vi "CSM - State Dashboard - DebugTool.vi"() -> ()   [LabVIEW 2017]
doc: "Real-time status dashboard for the entire CSM program module."
uses:
  user.lib/_NEVSTOP/Communicable State Machine(CSM)/_Support/Typedef/_CSM_GlobalLog_MSG.ctl
  user.lib/_NEVSTOP/Communicable State Machine(CSM)/_Support/Typedef/_CSM_Response Source Message.ctl
  user.lib/_NEVSTOP/Communicable State Machine(CSM)/_Support/Typedef/_CSM_GlobalLog_MSG_TYPE.ctl
  c0297aac-4a47-44f3-ae53-0a8cf90c2ba3.vi
  62af1497-def4-443f-94d3-5d00758f2f69.vi
  <vilib>/Utility/config.llb/Close Config Data.vi
  <vilib>/Utility/config.llb/Write Key.vi
  <vilib>/Utility/config.llb/Write Key (Double).vi
  <vilib>/Utility/config.llb/Write Key (I32).vi
  <vilib>/Utility/config.llb/Write Key (String).vi
  user.lib/_NEVSTOP/Communicable State Machine(CSM)/_csmHelper/lvcsmFile/Path to lvcsm String.vi
  <vilib>/Utility/config.llb/Remove Key.vi
  <vilib>/Utility/config.llb/Get Key Names.vi
  <vilib>/Utility/Data Type/Get Type Information.vi
  <vilib>/Utility/Data Type/Get Array Information.vi
  <vilib>/Utility/config.llb/Write Key (Boolean).vi
  <vilib>/Utility/config.llb/Open Config Data.vi
  user.lib/_NEVSTOP/Communicable State Machine(CSM)/_csmHelper/lvcsmFile/lvcsm File Path.vi
  user.lib/_NEVSTOP/Communicable State Machine(CSM)/_csmHelper/lvcsmFile/_Array of VData to VCluster.vi
  <vilib>/Utility/config.llb/Read Key.vi
  <vilib>/Utility/config.llb/Read Key (Double).vi
  <vilib>/Utility/config.llb/Read Key (I32).vi
  user.lib/_NEVSTOP/Communicable State Machine(CSM)/_csmHelper/lvcsmFile/lvcsm String to Path.vi
  <vilib>/Utility/config.llb/Read Key (String).vi
  <vilib>/Utility/config.llb/Read Key (Boolean).vi
  user.lib/_NEVSTOP/Communicable State Machine(CSM)/_Polymophic/Add State(s) to Queue By BOOL(Element).vi
  user.lib/_NEVSTOP/Communicable State Machine(CSM)/_tool/_ui/csm-ui-support.lvlib
  user.lib/_NEVSTOP/Communicable State Machine(CSM)/Communicable State Machine.lvlib
panel:
  in  "ColNum:":i16=4 min=2 max=10 step=1
  in  "RowNum:":i16=2 min=2 max=10 step=1
  in  "Clear CSM":bool
  out "Dashboard":T1(array[cluster])
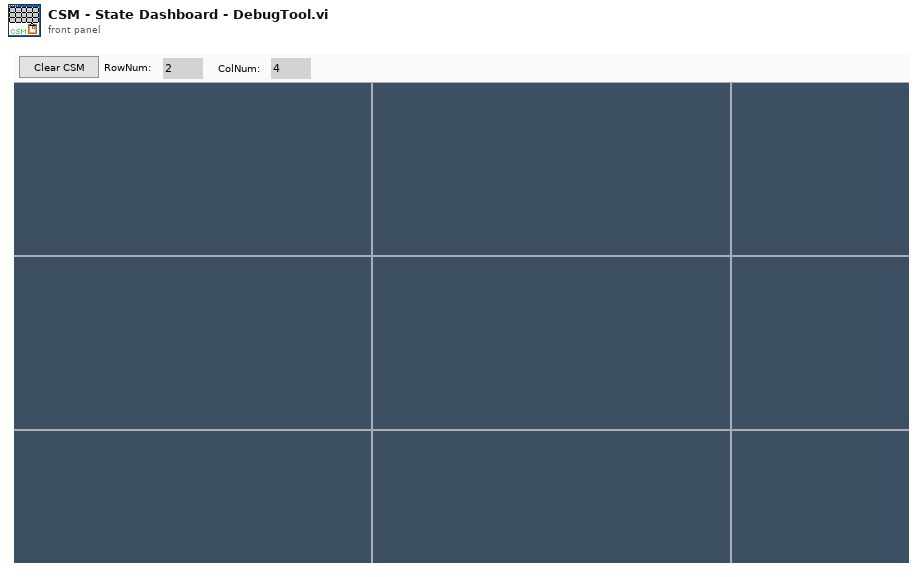
[diagram p1: front panel]
types:
  T1 = cluster{"Label":string, "Value":string, "String":string}[][]
  T2 = enum32{"Invalid", "Standard", "Closed", "Hidden", "Minimized", "Maximized"}
  T3 = enum32{"invalid app kind", "Development System", "Run Time System", "Student Edition", "Embedded LabVIEW", "Evaluation", "Custom"}
  T4 = typedef "Communicable State Machine.lvlib/_CSM_GlobalLog_MSG.ctl" = cluster{"Name (\"\" to Use UUID)":string, "Current State":string, "Arguments":string, "Source Message":T5, "Source Module":string, "Complete(T)/Start(F)":bool, "LogType":T6, "Time Stamp":timestamp}
  T5 = typedef "Communicable State Machine.lvlib/_CSM_Response Source Message.ctl" = cluster{"‘State":string, "’Arguments":string, "’Error":errorcluster}
  T6 = typedef "Communicable State Machine.lvlib/_CSM_GlobalLog_MSG_TYPE.ctl" = enum16{"User Log", "State Change", "Status", "Interrupt", "Register", "Unregister", "Error Log", "Module Created", "Module Destroyed"}
  T7 = cluster{"Label":string, "Value":string, "String":string}
  T8 = cluster{"Core":cluster{"Current VI Reference":refnum<vi>, "Close Panel on Exit?":bool}, "Global-DataTable":string[][], "Configuration":cluster{"NumRows":i16, "NumCols":i16}, "Global Log Event":refnum<user-event>, "Log":T4}
  T9 = cluster{"Current VI Reference":refnum<vi>, "Close Panel on Exit?":bool}
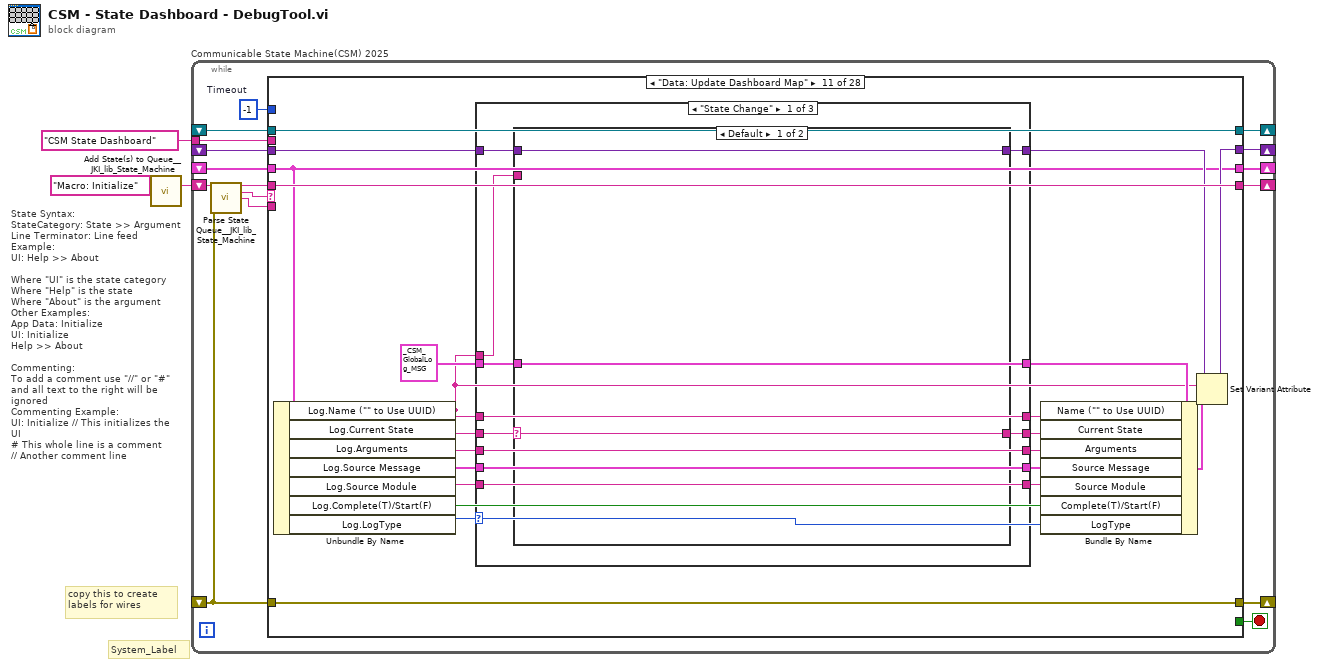
[diagram p0: block diagram]
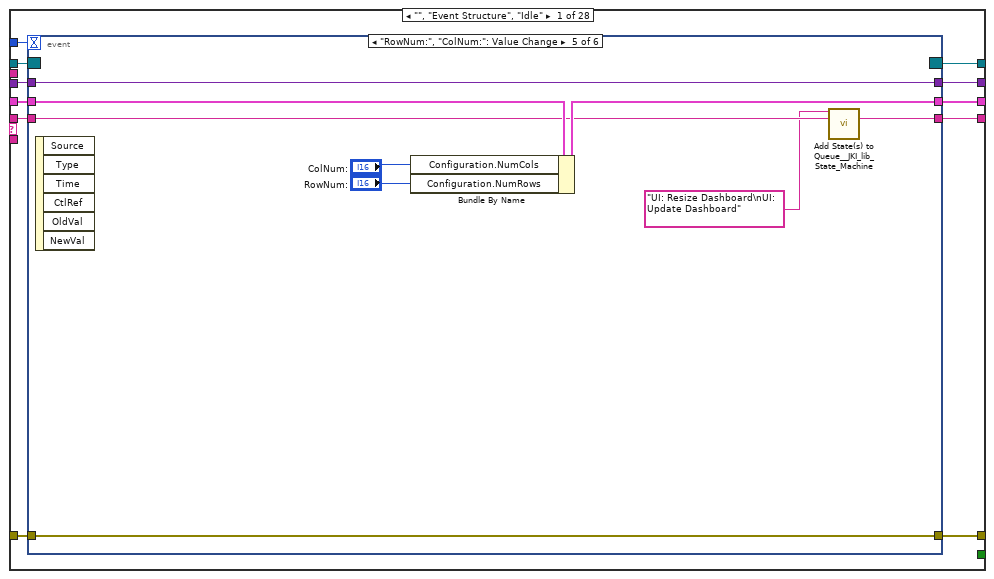
[diagram p2: hidden frame]
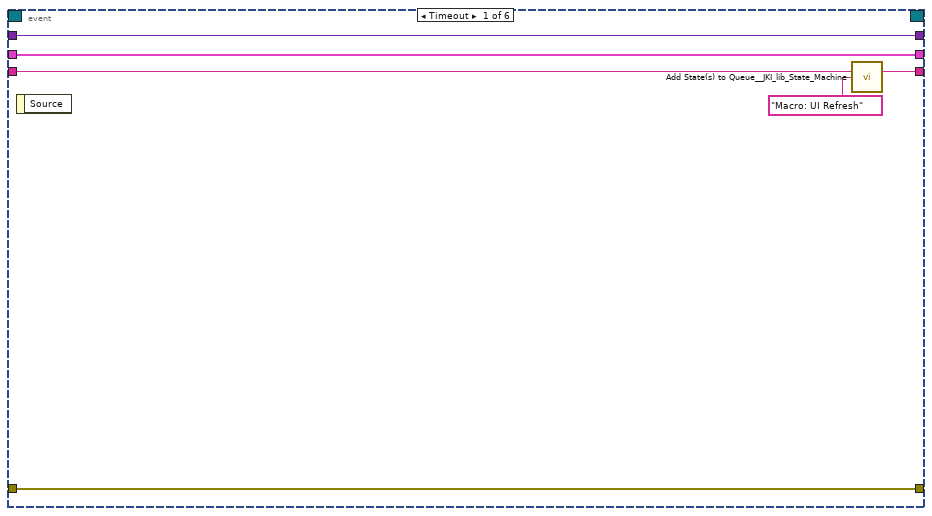
[diagram p3: hidden frame]
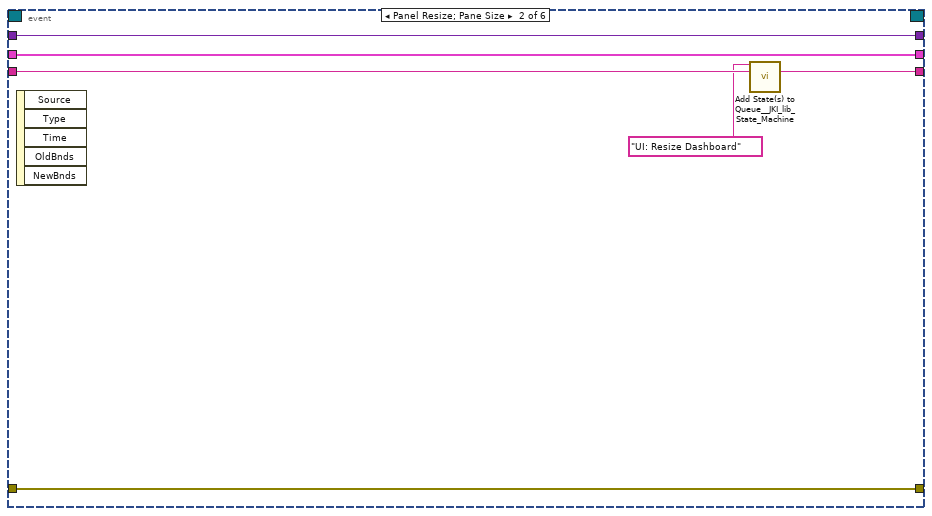
[diagram p4: hidden frame]
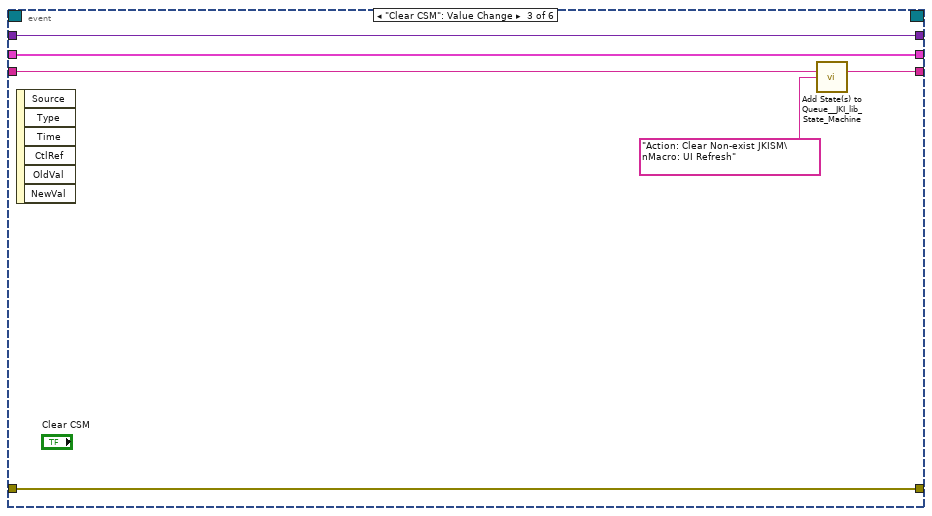
[diagram p5: hidden frame]
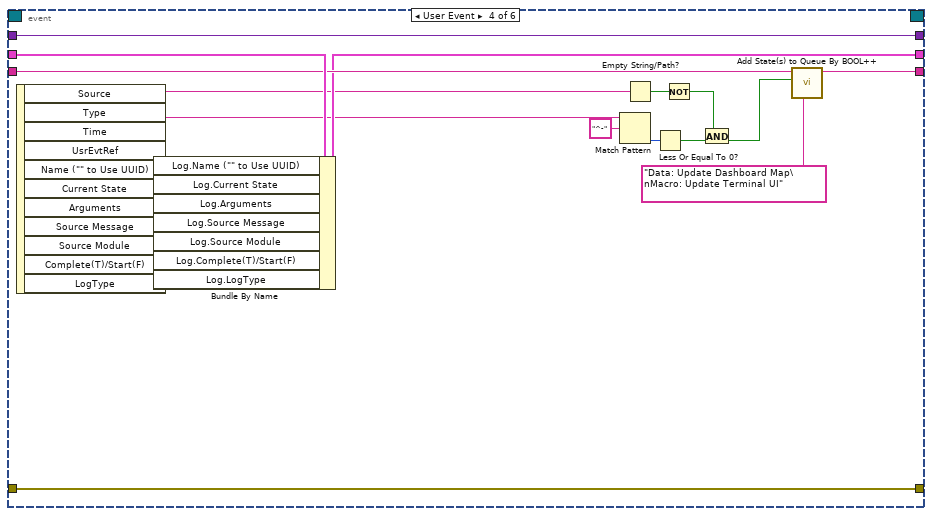
[diagram p6: hidden frame]
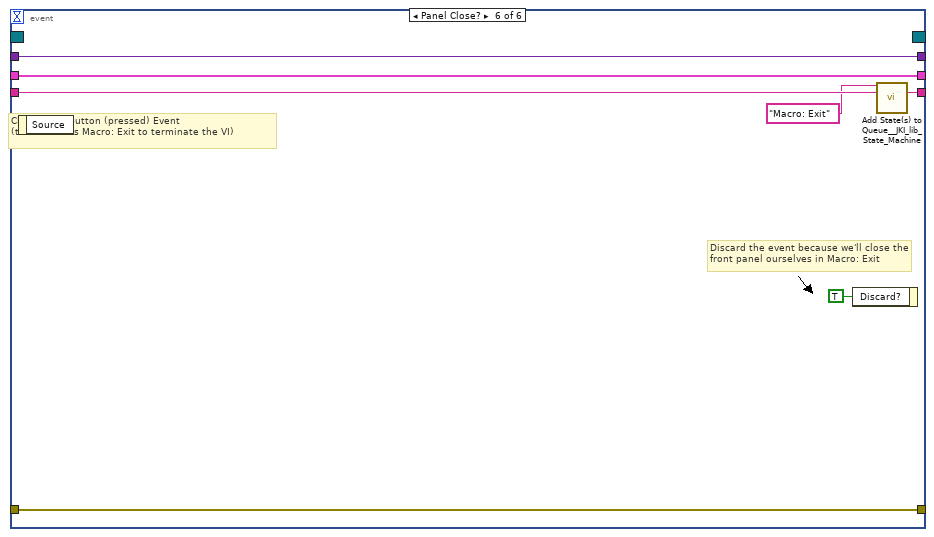
[diagram p7: hidden frame]
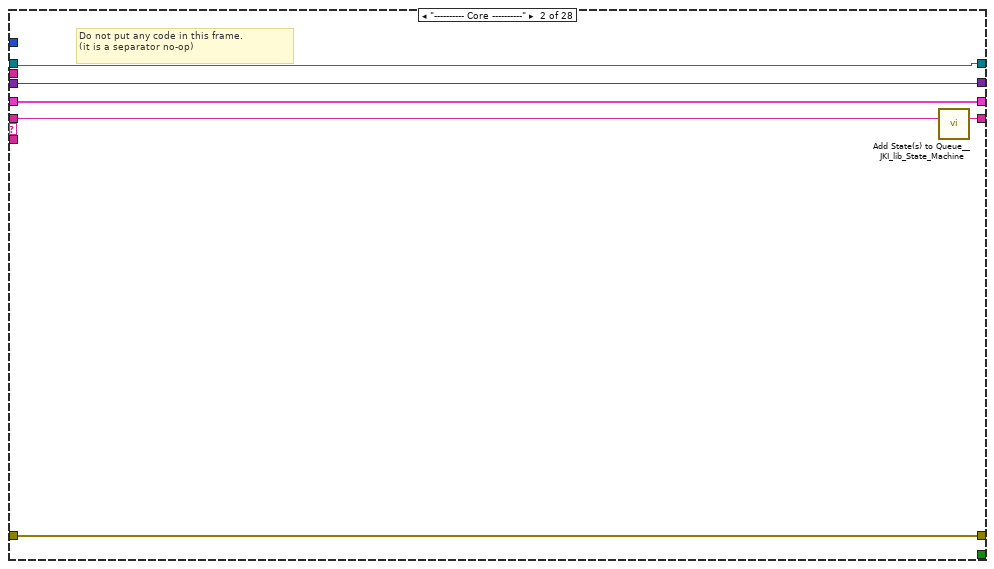
[diagram p8: hidden frame]
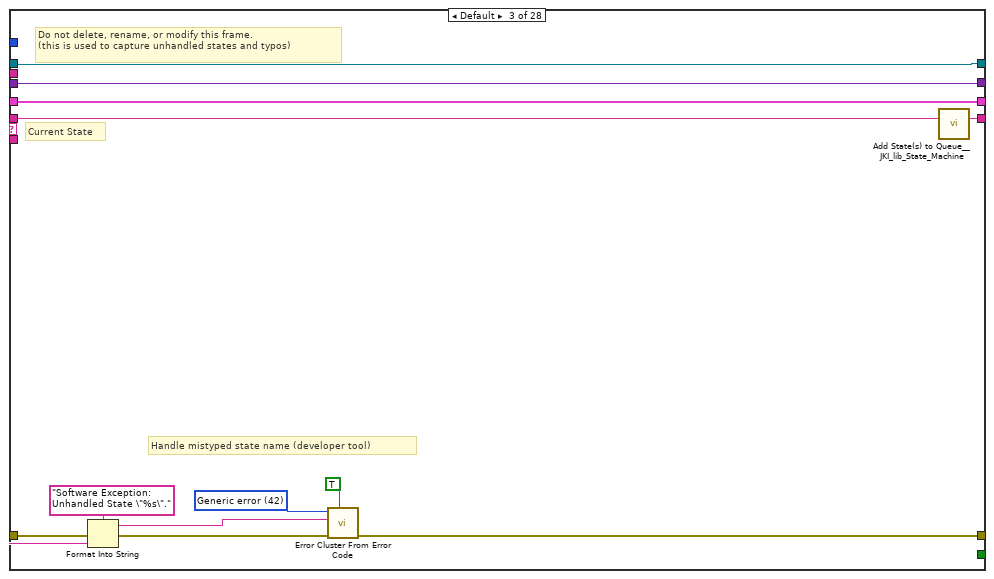
[diagram p9: hidden frame]
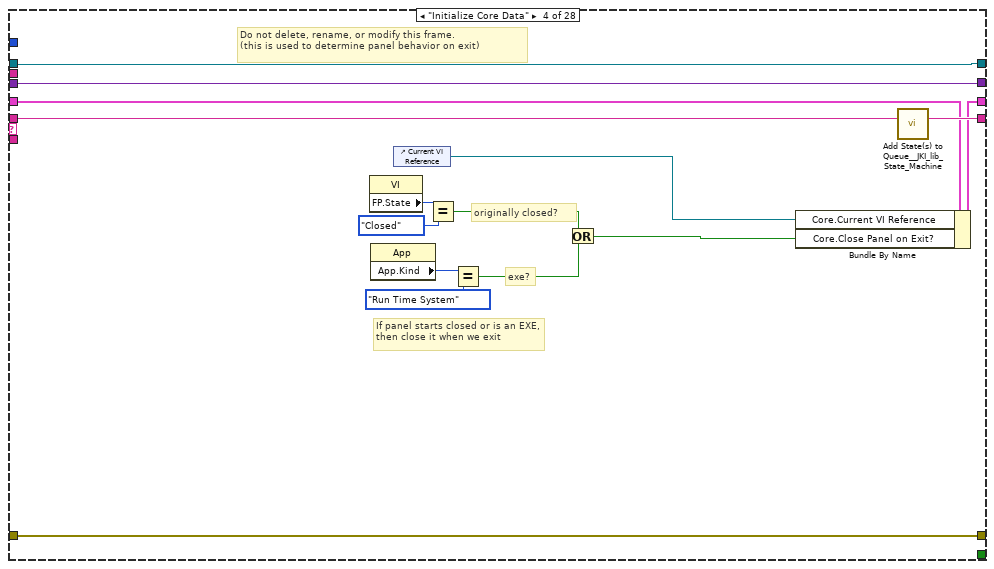
[diagram p10: hidden frame]
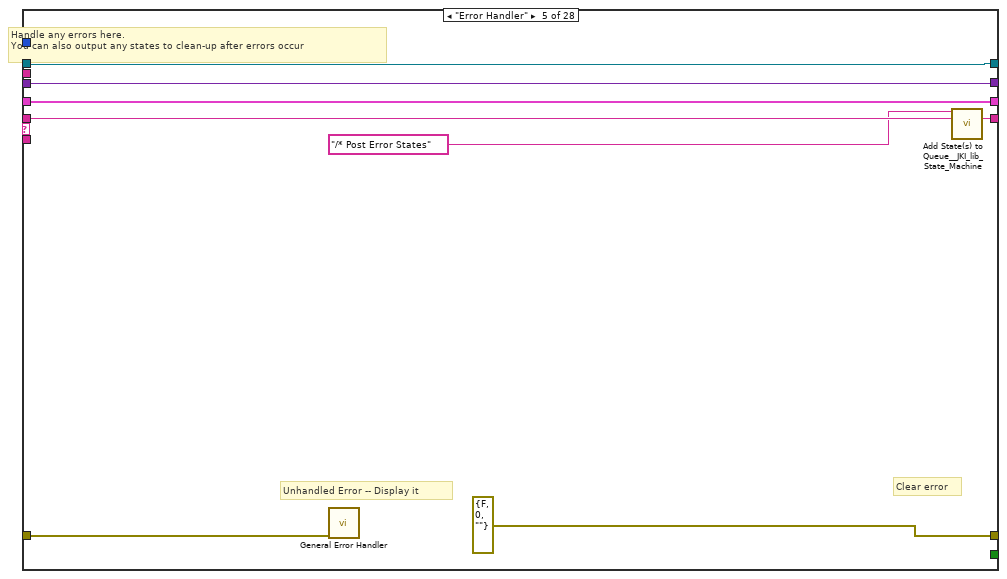
[diagram p11: hidden frame]
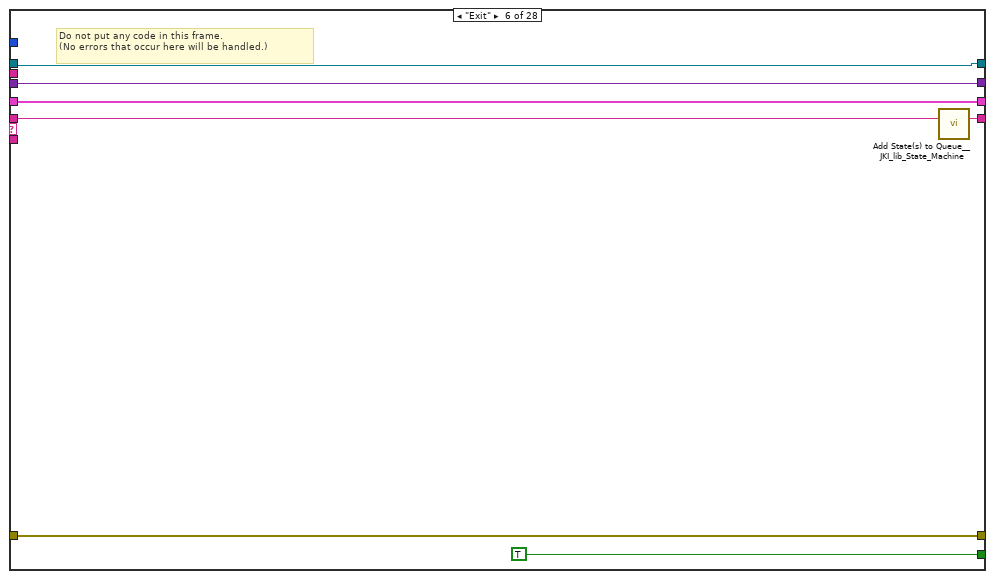
[diagram p12: hidden frame]
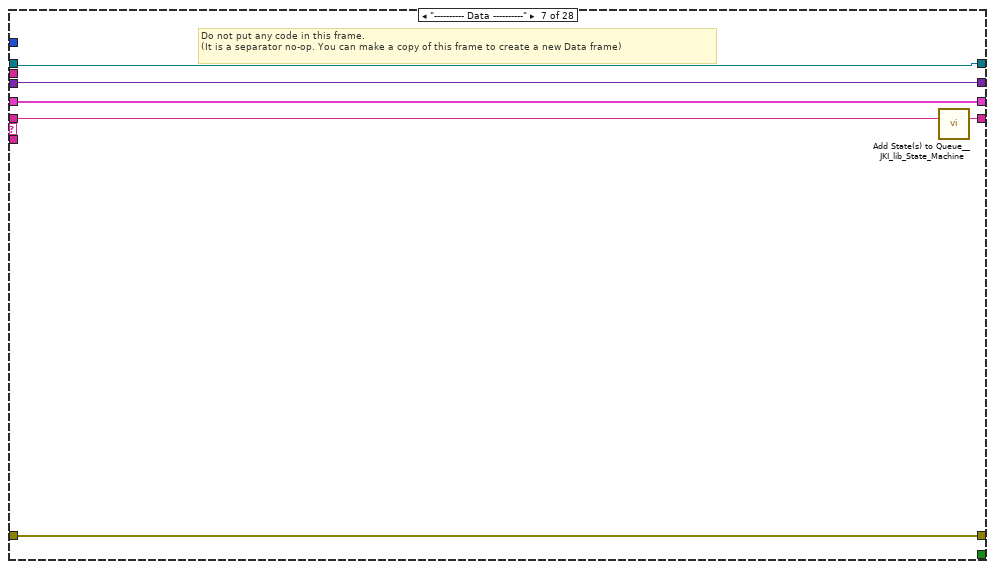
[diagram p13: hidden frame]
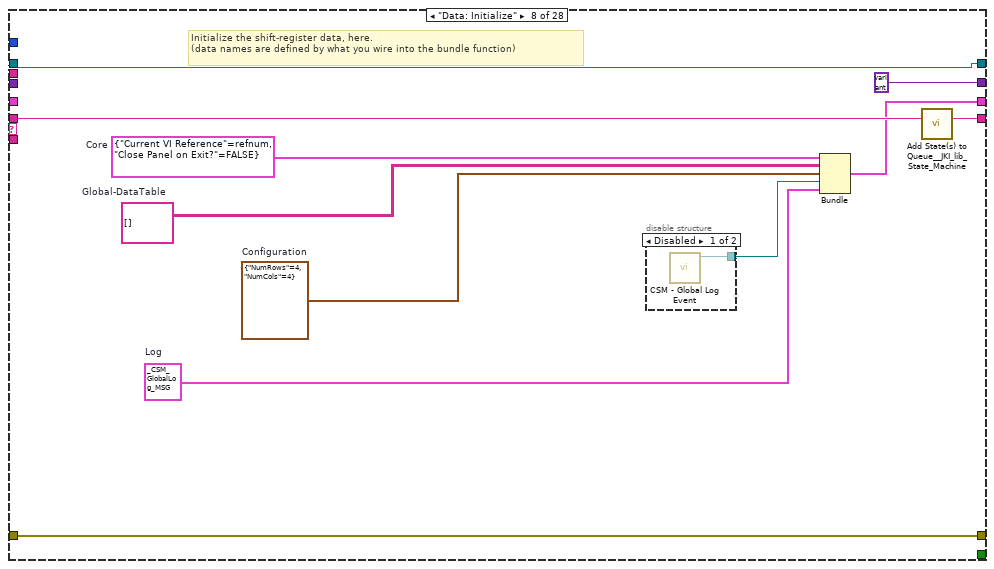
[diagram p14: hidden frame]
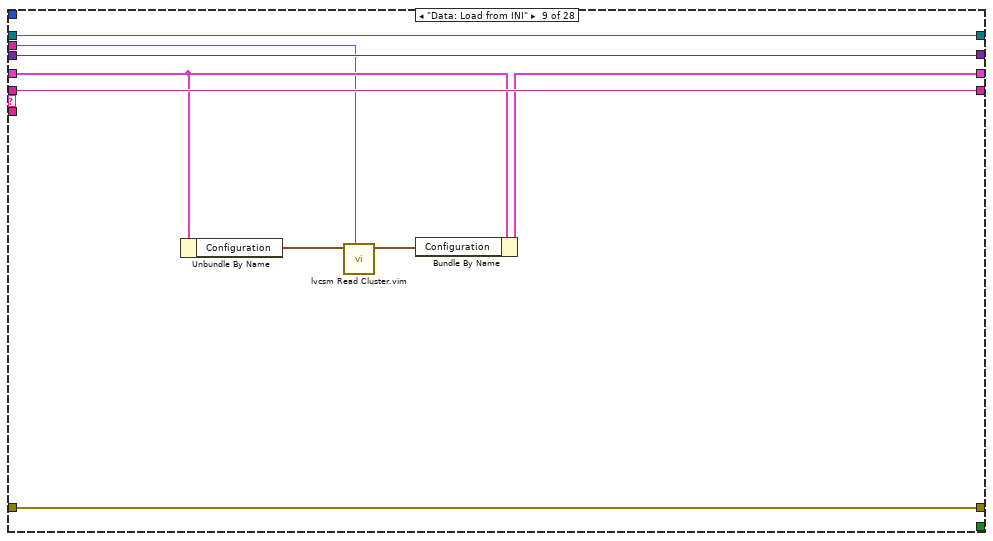
[diagram p16: hidden frame]
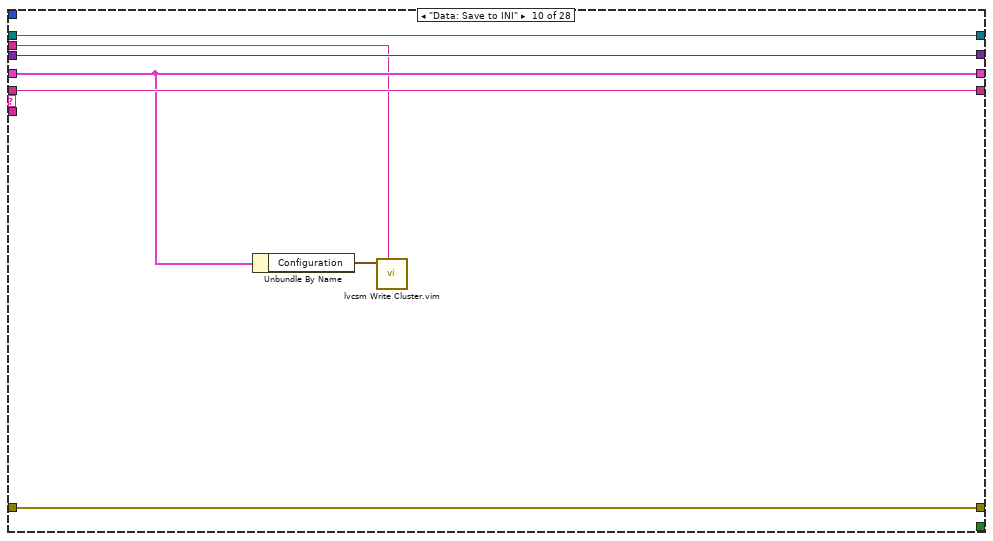
[diagram p17: hidden frame]
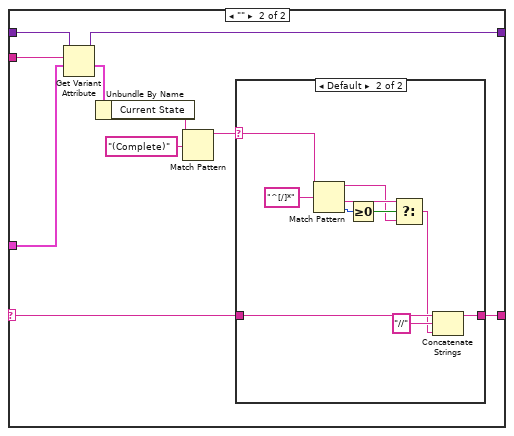
[diagram p18: hidden frame]
diagram:
  # "State Syntax:\nStateCategory: State >> Argument\nLine Terminator: Line feed\nExample:\nUI: Help >> About\n\nWhere \"UI\" is the state category\nWhere \"Help\" is the state\nWhere \"About\" is the argument\nOther Examples:\nApp Data: Initialize\nUI: Initialize\nHelp >> About\n\nCommenting:\nTo add a comment use \"//\" or \"#\" and all text to the right will be ignored\nCommenting Example:\nUI: Initialize // This initializes the UI\n# This whole line is a comment\n// Another comment line"
  # "copy this to create labels for wires"
  # "System_Label"
  n1 = call <vilib>:"Add State(s) to Queue__JKI_lib_State_Machine.vi"("State(s) in (\"\")"="Macro: Initialize") -> ("States Out"=w2:string)  [unwired: 14 in]
  n2 = while "Communicable State Machine(CSM) 2025" {
    shift-right: [w12] -> _
    shift-left: _ -> [w11]
    shift-right: [w15] -> _
    shift-left: _ -> [w9]
    shift-right: [w14] -> _
    shift-left: w2 -> [w16]
    shift-right: [w8] -> _
    shift-left: _ -> [w7]
    shift-right: [w6] -> _
    shift-left: _ -> [w5]
    tunnel: "CSM State Dashboard" ("Section") -> [w4]
    stop <- w13 stop-if-true
    w10 = -1  # Timeout
    n3 = call <vilib>:"Parse State Queue__JKI_lib_State_Machine.vi"("State Queue"=w16, "Error In (no error)"=w9) -> ("Remaining States"=w18:string, "Current State"=w19:string, "Arguments"=w17:string)  [unwired: 11 in]
    n4 = case shown="\"Data: Update Dashboard Map\"" w19 {
      selector: w19 -> [_ _ w93 _ _ _ _ _ _ _ _ _ _ _ _ _ _ _ _ _ _ _ _ _ _ _ _ _]
      tunnel: w18 -> [w30 w90 w97 w118 w126 w133 w139 w150 w159 w166 w188 w248 w254 w263 w275 w288 w365 w380 w390 w398 w406 w413 w420 w428 w435 w448 w452 w463]
      tunnel: w17 -> [_ _ _ _ _ _ _ _ _ _ _ _ _ _ w270 w282 _ _ _ _ _ _ _ _ _ _ _ _]
      tunnel: w11 -> [w28 w87 w95 w111 w123 w131 w136 _ w155 w163 w175 w243 w251 w259 w273 w284 w361 w377 w389 w397 w402 w410 w417 w423 w432 w445 w451 w462]
      tunnel: [w27 w88 w99 w115 errorcluster {"status"=FALSE, "code"=0, "source"=""} ("error out") w130 w137 w146 w160 w167 w189 w242 w252 w261 w271 w285 w362 w378 w391 w399 w407 w411 w418 w426 w433 w446 w453 w464] -> w15
      tunnel: w9 -> [w26 w88 w98 w115 w122 w130 w137 w146 w160 w167 w189 w245 w252 w261 w272 w286 _ w378 w391 w399 w407 w411 w418 w426 w433 w446 w453 w464]
      tunnel: [w29 w89 w96 w117 w125 w132 w138 w149 w159 w166 w188 w247 w253 w262 w274 w287 w364 w379 w390 w398 w406 w412 w419 w427 w434 w447 w452 w463] -> w14
      tunnel: [_ _ _ _ _ TRUE _ _ _ _ _ _ _ _ _ _ _ _ _ _ _ _ _ _ _ _ _ _] -> w13
      tunnel: [w25 w87 w95 w116 w123 w131 w136 w148 w156 w163 w175 w243 w251 w259 w273 w284 w361 w377 w389 w393 w402 w410 w417 w423 w432 w445 w451 w462] -> w12
      tunnel: w10 -> [w24 _ _ _ _ _ _ _ _ _ _ _ _ _ _ _ _ _ _ _ _ _ _ _ _ _ _ _]
      tunnel: [w22 w86 w92 w105 w120 w128 w135 variant w158 w165 w176 w241 w250 w256 w269 w281 w358 w372 w388 w396 w405 w409 w415 w422 w430 w438 w450 w458] -> w8
      tunnel: w7 -> [w23 w86 w92 w105 w120 w128 w135 _ w158 w165 w177 w241 w250 w256 w269 w281 w358 w371 w388 w396 w405 w409 w415 w422 w430 w438 w450 w460]
      tunnel: [w20 w85 w91 w104 w119 w127 w134 w143 w157 w164 w187 w240 w249 w255 w268 w280 w357 w368 w387 w394 w404 w408 w414 w421 w429 w437 w449 w461] -> w6
      tunnel: w5 -> [w21 w85 w91 w104 w119 w127 w134 w143 w157 w164 w187 w240 w249 w255 w268 w280 w357 w368 w387 _ w404 w408 w414 w421 w429 w437 w449 w461]
      tunnel: w4 -> [_ _ _ _ _ _ _ _ w154 w161 _ _ _ _ _ _ _ _ _ _ _ _ _ _ _ _ _ _]
      frame "", "Event Structure", "Idle" {
        n5 = event shown="[4] \"RowNum:\", \"ColNum:\": Value Change" {
          selector: w21 -> [_ _ _ _ _ _]
          dyn-events: [_ _ _ _ _ _] -> w20
          timeout: w24 -> [_ _ _ _ _ _]
          tunnel: w30 -> [w36 w39 w45 w63 w70 w84]
          tunnel: [w35 w40 w44 w67 w71 w83] -> w29
          tunnel: w28 -> [w33 w41 w47 w64 w76 w82]
          tunnel: [w34 w42 w48 w68 w77 w79] -> w27
          tunnel: w26 -> [w34 w42 w48 w68 w77 w79]
          tunnel: [w33 w41 w47 w62 w74 w82] -> w25
          tunnel: w23 -> [w31 w37 w46 w65 w75 w78]
          tunnel: [w31 w37 w46 w65 w75 w78] -> w22
          event Timeout {
            n6 = event-data() -> ()  [unwired: 1 in, 1 out]
            n7 = call <vilib>:"Add State(s) to Queue__JKI_lib_State_Machine.vi"("State(s) in (\"\")"=w36, "State(s) at Back (\"\")"="Macro: UI Refresh" ("State(s) in Front (\"\")")) -> ("States Out"=w35:string)  [unwired: 13 in]
          }
          event Panel Resize; Pane Size {
            n8 = event-data() -> ()  [unwired: 1 in, 5 out]
            n9 = call <vilib>:"Add State(s) to Queue__JKI_lib_State_Machine.vi"("State(s) in Front (\"\")"="UI: Resize Dashboard" ("State(s) in Front (\"\")"), "State(s) in (\"\")"=w39) -> ("States Out"=w40:string)  [unwired: 13 in]
          }
          event "Clear CSM": Value Change {
            n10 = event-data() -> ()  [unwired: 1 in, 6 out]
            n11 = call <vilib>:"Add State(s) to Queue__JKI_lib_State_Machine.vi"("State(s) in (\"\")"=w45, "State(s) at Back (\"\")"="Action: Clear Non-exist JKISM\nMacro: UI Refresh" ("State(s) at Back (\"\")")) -> ("States Out"=w44:string)  [unwired: 13 in]
          }
          event User Event {
            n12 = event-data() -> ("Name (\"\" to Use UUID)"=w51:string, "Current State"=w57:string, "Arguments"=w58:string, "Source Message"=w59:T5, "Source Module"=w60:string, "Complete(T)/Start(F)"=w61:bool, "LogType"=w56:T6)  [unwired: 1 in, 4 out]
            n13 = Bundle By Name(cluster=w64, "Log.Name (\"\" to Use UUID)"=w51, "Log.Current State"=w57, "Log.Arguments"=w58, "Log.Source Message"=w59, "Log.Source Module"=w60, "Log.Complete(T)/Start(F)"=w61, "Log.LogType"=w56) -> (w62:T8)
            n14 = Match Pattern(string=w51, regular expression="^-") -> (offset past match=w54:i32)  [unwired: 1 in, 3 out]
            n15 = Empty String/Path?(string/path=w51) -> (empty?=w50:bool)
            n16 = Less Or Equal To 0?(x=w54) -> (x <= 0?=w53:bool)
            n17 = Not(x=w50) -> (.not. x?=w49:bool)
            n18 = And(x=w49, y=w53) -> (x .and. y?=w52:bool)
            n19 = call-poly "Add State(s) to Queue By BOOL++.vi"("TRUE (\"\")"="Data: Update Dashboard Map\nMacro: Update Terminal UI" ("State(s) at Back (\"\")"), "Condition"=w52, "State Queue (\"\")"=w63) -> ("Remaining States"=w67:string)  [unwired: 8 in]
          }
          event "RowNum:", "ColNum:": Value Change {
            n20 = event-data() -> ()  [unwired: 1 in, 6 out]
            n21 = Bundle By Name(cluster=w76, "Configuration.NumCols"="ColNum:", "Configuration.NumRows"="RowNum:") -> (w74:T8)
            n22 = call <vilib>:"Add State(s) to Queue__JKI_lib_State_Machine.vi"("State(s) in Front (\"\")"="UI: Resize Dashboard\nUI: Update Dashboard" ("State(s) in Front (\"\")"), "State(s) in (\"\")"=w70) -> ("States Out"=w71:string)  [unwired: 13 in]
          }
          event Panel Close? {
            # "Discard the event because we'll close the front panel ourselves in Macro: Exit"
            # "Close Panel button (pressed) Event\n(this executes Macro: Exit to terminate the VI)"
            n23 = event-data() -> ()  [unwired: 1 in, 1 out]
            n24 = event-data("Discard?"=TRUE) -> ()  [unwired: 1 in, 1 out]
            n25 = call <vilib>:"Add State(s) to Queue__JKI_lib_State_Machine.vi"("State(s) in Front (\"\")"="Macro: Exit", "State(s) in (\"\")"=w84) -> ("States Out"=w83:string)  [unwired: 13 in]
          }
        }
      }
      frame "---------- Core ----------" {
        # "Do not put any code in this frame.\n(it is a separator no-op)"
        n26 = call <vilib>:"Add State(s) to Queue__JKI_lib_State_Machine.vi"("State(s) in (\"\")"=w90) -> ("States Out"=w89:string)  [unwired: 14 in]
      }
      frame Default {
        w102 = 42 items=["No error", "Argument error", "Memory is full", "Out of zone", "End of file", "File already open", "Generic file I/O error", "File not found", "File permission error", "Disk is full", "Duplicate path", "Too many files open", "System feature not enabled", "Resource file not found", "Cannot add resource", "Resource not found", "Image not found", "Image memory error", "Pen does not exist", "Config type invalid", "Config token not found", "Config parse error", "Config memory error", "Bad external code format", "Bad external code offset", "External code not present", "Null window", "Destroy window error", "Null menu", "Print aborted", "Bad print record", "Print driver error", "Windows error during printing", "Memory error during printing", "Print dialog error", "Generic print error", "Invalid device refnum", "Device not found", "Device parameter error", "Device unit error", "Cannot open device", "Device call aborted", "Generic error", "Cancelled by user", "Object ID too low", "Object ID too high", "Object not in heap", "Unknown heap", "Unknown object (invalid DefProc)", "Unknown object (DefProc not in table)", "Message out of range", "Invalid (null) method", "Unknown message", "Manager call not supported", "Bad address", "Network operation in progress", "Network operation timed out", "Connection is busy", "Network attribute not supported", "Network error", "Address in use", "System out of memory", "Connection aborted", "Connection refused", "Not connected", "Already connected", "Connection closed", "Initialization error (interapplication manager)", "Bad occurrence", "Wait on unbound occurrence handler", "Occurrence queue overflow", "Datalog type conflict", "Unused", "Unrecognized type (interapplication manager)", "Memory corrupt", "Failed to make temporary DLL", "Old CIN version", "Drag socket not found", "Failed to load drop-object", "Failed to register OLE object", "Failed to release OLE object", "Format specifier type mismatch", "Unknown format specifier", "Too few format specifiers", "Too many format specifiers", "Scan failed", "Newer CIN version", "Error converting to variant", "Runtime menu error", "Password tampered", "Variant attribute not found", "Incompatible variant data type", "Event data is not available", "Event Store is not present", "Occurrence is not found", "Event Queue is not created", "Event info is not available", "Refnum passed is NULL", "Error retrieving Class GUID", "Error retrieving CoClass GUID", "Error retrieving TypeLib GUID.", "Bad built application magic bytes.", "Specific driver is different from the specific driver associated with the Logical Name.", "There is no session opened to the class driver.", "Max Error", "MAX - Error with config objects", "MAX - Error loading configuration", "MAX - Group not supported"]
        # "Current State"
        # "Do not delete, rename, or modify this frame.\n(this is used to capture unhandled states and typos)"
        # "Handle mistyped state name (developer tool)"
        n27 = Format Into String(format string="Software Exception: Unhandled State \"%s\"." ("message"), error in=w98, w93) -> (resulting string=w101:string, error out=w100:errorcluster)  [unwired: 1 in]
        n28 = call <vilib>:"Error Cluster From Error Code.vi"("show call chain? (False)"=TRUE, "error in (no error)"=w100, "error message (\"\")"=w101, "error code (0)"=w102) -> ("error out"=w99:errorcluster)  [unwired: 5 in]
        n29 = call <vilib>:"Add State(s) to Queue__JKI_lib_State_Machine.vi"("State(s) in (\"\")"=w97) -> ("States Out"=w96:string)  [unwired: 14 in]
      }
      frame "Initialize Core Data" {
        # "Do not delete, rename, or modify this frame.\n(this is used to determine panel behavior on exit)"
        # "originally closed?"
        # "exe?"
        # "If panel starts closed or is an EXE, then close it when we exit"
        n30 = property class="VI"() -> ("FP.State"=w108:T2)  [unwired: 2 in, 2 out]
        n31 = property class="App"() -> ("App.Kind"=w114:T3)  [unwired: 2 in, 2 out]
        n32 = control-ref of="Current VI Reference"() -> (w109:refnum<vi>)
        n33 = Equal?(x=w108, y=T2."Closed" ("Front Panel Window:State")) -> (x = y?=w106:bool)
        n34 = Equal?(x=w114, y=T3."Run Time System" ("Application:Kind")) -> (x = y?=w112:bool)
        n35 = Or(x=w106, y=w112) -> (x .or. y?=w110:bool)
        n36 = Bundle By Name(cluster=w111, "Core.Current VI Reference"=w109, "Core.Close Panel on Exit?"=w110) -> (w116:T8)
        n37 = call <vilib>:"Add State(s) to Queue__JKI_lib_State_Machine.vi"("State(s) in (\"\")"=w118) -> ("States Out"=w117:string)  [unwired: 14 in]
      }
      frame "Error Handler" {
        # "Unhandled Error -- Display it"
        # "Handle any errors here.\nYou can also output any states to clean-up after errors occur"
        # "Clear error"
        n38 = call <vilib>:"General Error Handler.vi"("error in (no error)"=w122) -> ()  [unwired: 10 in, 5 out]
        n39 = call <vilib>:"Add State(s) to Queue__JKI_lib_State_Machine.vi"("State(s) in Front (\"\")"="/* Post Error States", "State(s) in (\"\")"=w126) -> ("States Out"=w125:string)  [unwired: 13 in]
      }
      frame "Exit" {
        # "Do not put any code in this frame.\n(No errors that occur here will be handled.)"
        n40 = call <vilib>:"Add State(s) to Queue__JKI_lib_State_Machine.vi"("State(s) in (\"\")"=w133) -> ("States Out"=w132:string)  [unwired: 14 in]
      }
      frame "---------- Data ----------" {
        # "Do not put any code in this frame.\n(It is a separator no-op. You can make a copy of this frame to create a new Data frame)"
        n41 = call <vilib>:"Add State(s) to Queue__JKI_lib_State_Machine.vi"("State(s) in (\"\")"=w139) -> ("States Out"=w138:string)  [unwired: 14 in]
      }
      frame "Data: Initialize" {
        w140 = cluster{"NumRows":i16, "NumCols":i16} {"NumRows"=4, "NumCols"=4}  # Configuration
        w141 = T4 {"Name (\"\" to Use UUID)"="", "Current State"="", "Arguments"="", "Source Message"={"‘State"="", "’Arguments"="", "’Error"={"status"=FALSE, "code"=0, "source"=""}}, "Source Module"="", "Complete(T)/Start(F)"=FALSE, "LogType"=enum."User Log", "Time Stamp"=timestamp(0 s since 1904-01-01)}  # Log
        w145 = string[][] []  # Global-DataTable
        w147 = T9 {"Current VI Reference"=refnum, "Close Panel on Exit?"=FALSE}  # Core
        # "Initialize the shift-register data, here.\n(data names are defined by what you wire into the bundle function)"
        n42 = disable-structure shown="Disabled" {
          disable-tunnel: [w151 _] -> w142
          frame Disabled {
            n43 = call "CSM - Global Log Event.vi"() -> ("Global Log Event"=w151:refnum<user-event>)  [unwired: 10 in, 1 out]
          }
          frame Enabled {
          }
        }
        n44 = Bundle("Core"=w147, "Global-DataTable"=w145, "Configuration"=w140, "Global Log Event"=w142, "Log"=w141) -> (w148:T8)  [unwired: 1 in]
        n45 = call <vilib>:"Add State(s) to Queue__JKI_lib_State_Machine.vi"("State(s) in (\"\")"=w150) -> ("States Out"=w149:string)  [unwired: 14 in]
      }
      frame "Data: Load from INI" {
        n46 = Unbundle By Name(w155) -> ("Configuration"=w153:cluster{"NumRows":i16, "NumCols":i16})
        n47 = call "lvcsm Read Cluster.vim"("Section"=w154, "Default Prototype"=w153) -> ("Cluster (Dup)"=w152:cluster{"NumRows":i16, "NumCols":i16})  [unwired: 8 in, 1 out]
        n48 = Bundle By Name(cluster=w155, "Configuration"=w152) -> (w156:T8)
      }
      frame "Data: Save to INI" {
        n49 = Unbundle By Name(w163) -> ("Configuration"=w162:cluster{"NumRows":i16, "NumCols":i16})
        n50 = call "lvcsm Write Cluster.vim"("Section"=w161, "Configuration"=w162) -> ()  [unwired: 9 in, 1 out]
      }
      frame "Data: Update Dashboard Map" {
        n51 = Unbundle By Name(w175) -> ("Log.Name (\"\" to Use UUID)"=w170:string, "Log.Current State"=w174:string, "Log.Arguments"=w173:string, "Log.Source Message"=w172:T5, "Log.Source Module"=w171:string, "Log.Complete(T)/Start(F)"=w168:bool, "Log.LogType"=w169:T6)
        n52 = case shown="\"State Change\"" w169 {
          tunnel: w177 -> [w195 w225 w239]
          tunnel: [w194 w225 w238] -> w185
          tunnel: T4 {"Name (\"\" to Use UUID)"="", "Current State"="", "Arguments"="", "Source Message"={"‘State"="", "’Arguments"="", "’Error"={"status"=FALSE, "code"=0, "source"=""}}, "Source Module"="", "Complete(T)/Start(F)"=FALSE, "LogType"=enum."User Log", "Time Stamp"=timestamp(0 s since 1904-01-01)} ("Cross JKI State Machine Data") -> [w192 w224 w237]
          tunnel: w170 -> [w193 _ w236]
          tunnel: w171 -> [w199 w229 _]
          tunnel: [w199 w229 w235] -> w183
          tunnel: w172 -> [w198 w228 _]
          tunnel: [w198 w228 w234] -> w182
          tunnel: w173 -> [w197 w227 _]
          tunnel: [w197 w227 w233] -> w181
          tunnel: w174 -> [w191 w223 _]
          tunnel: [w190 w223 w230] -> w180
          tunnel: w170 -> [w196 w226 _]
          tunnel: [w196 w226 w231] -> w179
          tunnel: [w192 w224 w232] -> w178
          frame "State Change" {
            n53 = case shown="Default" w191 {
              selector: w191 -> [w200 w203]
              tunnel: w195 -> [w201 w211]
              tunnel: [w201 w210] -> w194
              tunnel: w193 -> [_ w209]
              tunnel: w192 -> [_ w207]
              tunnel: [w200 w202] -> w190
              frame Default {
              }
              frame "" {
                n54 = Get Variant Attribute(Variant=w211, name=w209, default value (empty Variant)=w207) -> (duplicate Variant=w210:variant, value=w208:T4)  [unwired: 1 in, 2 out]
                n55 = Unbundle By Name(w208) -> ("Current State"=w206:string)
                n56 = Match Pattern(string=w206, regular expression="(Complete)") -> (before substring=w204:string)  [unwired: 1 in, 3 out]
                n57 = case shown="Default" w204 {
                  selector: w204 -> [_ w218]
                  tunnel: w203 -> [w212 w222]
                  tunnel: [w212 w221] -> w202
                  frame "" {
                  }
                  frame Default {
                    n58 = Match Pattern(string=w218, regular expression="^[/]*") -> (before substring=w213:string, after substring=w215:string, offset past match=w217:i32)  [unwired: 1 in, 1 out]
                    n59 = Greater Or Equal To 0?(x=w217) -> (x >= 0?=w216:bool)
                    n60 = Select(t=w215, s=w216, f=w213) -> (s? t:f=w214:string)
                    n61 = Concatenate Strings(w222, "//" ("string"), w214) -> (w221:string)
                  }
                }
              }
            }
          }
          frame "Error Log" {
          }
          frame Default {
            n62 = Get Variant Attribute(Variant=w239, name=w236, default value (empty Variant)=w237) -> (duplicate Variant=w238:variant, value=w232:T4)  [unwired: 1 in, 2 out]
            n63 = Unbundle By Name(w232) -> ("Name (\"\" to Use UUID)"=w231:string, "Current State"=w230:string, "Arguments"=w233:string, "Source Message"=w234:T5, "Source Module"=w235:string)
          }
        }
        n64 = Bundle By Name(cluster=w178, "Name (\"\" to Use UUID)"=w179, "Current State"=w180, "Arguments"=w181, "Source Message"=w182, "Source Module"=w183, "Complete(T)/Start(F)"=w168, "LogType"=w169) -> (w186:T4)
        n65 = Set Variant Attribute(Variant=w185, name=w170, value=w186) -> (Variant out=w176:variant)  [unwired: 1 in, 2 out]
      }
      frame "Data: Cleanup" {
        # "Cleanup any data and references, here.\n(this is called automatically, by the Macro: Exit)"
        n66 = Unbundle By Name(w243) -> ("Core.Current VI Reference"=w246:refnum<vi>)
        n67 = Close Reference(reference=w246, error in (no error)=w245) -> (error out=w244:errorcluster)
        n68 = Merge Errors(w244) -> (w242:errorcluster)
        n69 = call <vilib>:"Add State(s) to Queue__JKI_lib_State_Machine.vi"("State(s) in (\"\")"=w248) -> ("States Out"=w247:string)  [unwired: 14 in]
      }
      frame "---------- UI ----------" {
        # "Do not put any code in this frame.\n(It is a separator no-op. You can make a copy of this frame to create a new UI frame)"
        n70 = call <vilib>:"Add State(s) to Queue__JKI_lib_State_Machine.vi"("State(s) in (\"\")"=w254) -> ("States Out"=w253:string)  [unwired: 14 in]
      }
      frame "UI: Initialize" {
        # "Initialize the User Interface, here.\n(this is called automatically, by the Macro: Init)"
        n71 = invoke class="VI" method="Default Vals.Reinit All"() -> (error out=w260:errorcluster)  [unwired: 3 in, 2 out]
        n72 = Unbundle By Name(w259) -> ("Configuration.NumRows"=w258:i16, "Configuration.NumCols"=w257:i16)
        n73 = flat-sequence {
          tunnel: w260 -> [_]
          tunnel: w258 -> [w265]
          tunnel: w257 -> [w264]
          frame #0 {
            n74 = Initialize Array(T7 {"Label"="", "Value"="", "String"=""} ("Dashboard"), w265, w264) -> (w266:T1)
            n75 = local write "RowNum:"(w265) -> ()
            n76 = local write "Dashboard"(w266) -> ()
            n77 = local write "ColNum:"(w264) -> ()
          }
        }
        n78 = call <vilib>:"Add State(s) to Queue__JKI_lib_State_Machine.vi"("State(s) in (\"\")"=w263) -> ("States Out"=w262:string)  [unwired: 14 in]
      }
      frame "UI: Cursor Set" {
        # "Argument"
        # "Set and Unset Cursor Busy.\n(Usage: \"UI: Cursor Set >> Busy|Idle\")"
        n79 = case shown="\"Idle\", Default" w270 {
          tunnel: w272 -> [w277 w279]
          tunnel: [w276 w278] -> w271
          frame "Idle", Default {
            n80 = call <vilib>:"Unset Busy.vi"("error in (no error)"=w277) -> ("error out"=w276:errorcluster)  [unwired: 10 in]
          }
          frame "Busy" {
            n81 = call <vilib>:"Set Busy.vi"("error in (no error)"=w279) -> ("error out"=w278:errorcluster)  [unwired: 9 in, 1 out]
          }
        }
        n82 = call <vilib>:"Add State(s) to Queue__JKI_lib_State_Machine.vi"("State(s) in (\"\")"=w275) -> ("States Out"=w274:string)  [unwired: 14 in]
      }
      frame "UI: Front Panel State" {
        # "Argument"
        # "Set Front Panel Open or Closed\n(Usage: \"UI: Front Panel State >> Open|Close\")"
        n83 = Unbundle By Name(w284) -> ("Core.Current VI Reference"=w283:refnum<vi>)
        n84 = case shown="\"Minimize\", \"Minimized\"" w282 {
          tunnel: w286 -> [w294 w309 w320 w333 w346]
          tunnel: [w296 w310 w322 w335 w348] -> w285
          tunnel: w283 -> [w295 w307 w321 w334 w347]
          frame "Open", "Standard", Default {
            w289 = T2."Standard" ("State")
            n85 = property class="VI"(reference=w295, error in=w294) -> (reference out=w292:refnum<vi>, error out=w293:errorcluster, "FP.State"=w291:T2)
            n86 = Not Equal?(x=w291, y=w289) -> (x != y?=w290:bool)
            n87 = case shown="True" w290 {
              tunnel: [w300 w302] -> w296
              tunnel: w293 -> [w299 w302]
              tunnel: w292 -> [w298 _]
              tunnel: w289 -> [w297 _]
              frame True {
                n88 = invoke class="VI" method="FP.Open"(reference=w298, error in=w299, "Activate"=TRUE, "State"=w297) -> (error out=w300:errorcluster)  [unwired: 1 in, 4 out]
              }
              frame False {
              }
            }
          }
          frame "Close", "Closed" {
            n89 = property class="VI"(reference=w307, error in=w309) -> (reference out=w306:refnum<vi>, error out=w308:errorcluster, "FP.State"=w304:T2)
            n90 = Not Equal?(x=w304, y=T2."Closed" ("Front Panel Window:State")) -> (x != y?=w303:bool)
            n91 = case shown="True" w303 {
              tunnel: [w311 w314] -> w310
              tunnel: w308 -> [w311 w313]
              tunnel: w306 -> [_ w312]
              frame False {
              }
              frame True {
                n92 = invoke class="VI" method="FP.Close"(reference=w312, error in=w313) -> (error out=w314:errorcluster)  [unwired: 1 in, 2 out]
              }
            }
          }
          frame "Hidden", "Hide" {
            w315 = T2."Hidden" ("State")
            n93 = property class="VI"(reference=w321, error in=w320) -> (reference out=w318:refnum<vi>, error out=w319:errorcluster, "FP.State"=w317:T2)
            n94 = Not Equal?(x=w317, y=w315) -> (x != y?=w316:bool)
            n95 = case shown="True" w316 {
              tunnel: [w326 w327] -> w322
              tunnel: w319 -> [w325 w327]
              tunnel: w318 -> [w324 _]
              tunnel: w315 -> [w323 _]
              frame True {
                n96 = invoke class="VI" method="FP.Open"(reference=w324, error in=w325, "State"=w323) -> (error out=w326:errorcluster)  [unwired: 2 in, 4 out]
              }
              frame False {
              }
            }
          }
          frame "Minimize", "Minimized" {
            w328 = T2."Minimized" ("State")
            n97 = property class="VI"(reference=w334, error in=w333) -> (reference out=w331:refnum<vi>, error out=w332:errorcluster, "FP.State"=w330:T2)
            n98 = Not Equal?(x=w330, y=w328) -> (x != y?=w329:bool)
            n99 = case shown="True" w329 {
              tunnel: [w339 w340] -> w335
              tunnel: w332 -> [w338 w340]
              tunnel: w331 -> [w337 _]
              tunnel: w328 -> [w336 _]
              frame True {
                n100 = invoke class="VI" method="FP.Open"(reference=w337, error in=w338, "State"=w336) -> (error out=w339:errorcluster)  [unwired: 2 in, 4 out]
              }
              frame False {
              }
            }
          }
          frame "Maximize", "Maximized" {
            w341 = T2."Maximized" ("State")
            n101 = property class="VI"(reference=w347, error in=w346) -> (reference out=w344:refnum<vi>, error out=w345:errorcluster, "FP.State"=w343:T2)
            n102 = Not Equal?(x=w343, y=w341) -> (x != y?=w342:bool)
            n103 = case shown="True" w342 {
              tunnel: [w352 w353] -> w348
              tunnel: w345 -> [w351 w353]
              tunnel: w344 -> [w350 _]
              tunnel: w341 -> [w349 _]
              frame True {
                n104 = invoke class="VI" method="FP.Open"(reference=w350, error in=w351, "State"=w349) -> (error out=w352:errorcluster)  [unwired: 2 in, 4 out]
              }
              frame False {
              }
            }
          }
        }
        n105 = call <vilib>:"Add State(s) to Queue__JKI_lib_State_Machine.vi"("State(s) in (\"\")"=w288) -> ("States Out"=w287:string)  [unwired: 14 in]
      }
      frame "UI: Resize Dashboard" {
        # "Do not put any code in this frame.\n(It is a separator no-op. You can make a copy of this frame to create a new UI frame)"
        n106 = control-ref of="Pane"() -> (w354:refnum<vi>)
        n107 = control-ref of="Dashboard"() -> (w363:refnum<vi>)
        n108 = Unbundle By Name(w361) -> ("Configuration.NumCols"=w359:i16, "Configuration.NumRows"=w360:i16)
        n109 = property class="Pane"(reference=w354) -> ("Width"=w356:u32, "Height"=w355:u32)  [unwired: 1 in, 2 out]
        n110 = call "Dashboard Cell2 Array Resize.vi"("Num Columns"=w359, "Num Rows"=w360, "Area Height"=w355, "Area Width"=w356, "Array 2"=w363) -> ("error out"=w362:errorcluster)  [unwired: 6 in]
        n111 = call <vilib>:"Add State(s) to Queue__JKI_lib_State_Machine.vi"("State(s) in (\"\")"=w365) -> ("States Out"=w364:string)  [unwired: 14 in]
      }
      frame "UI: Update Dashboard" {
        # "Do not put any code in this frame.\n(It is a separator no-op. You can make a copy of this frame to create a new UI frame)"
        n112 = Get Variant Attribute(Variant=w371) -> (duplicate Variant=w372:variant, names=w370:string[], values=w369:variant[])  [unwired: 3 in, 1 out]
        n113 = Variant To Data(type=T4[] [], Variant=w369) -> (data=w366:T4[])  [unwired: 1 in, 1 out]
        n114 = for {
          tunnel: w370 -> [w385] mode=indexing
          tunnel: [w384] -> w376 mode=indexing
          tunnel: w366 -> [w383] mode=indexing
          n115 = Unbundle By Name(w383) -> ("Current State"=w382:string, "Arguments"=w381:string)  [unwired: 1 out]
          n116 = Bundle By Name(cluster=T7 {"Label"="", "Value"="", "String"=""}, "Label"=w385, "Value"=w382, "String"=w381) -> (w384:T7)
        }
        n117 = Unbundle By Name(w377) -> ("Configuration.NumRows"=w374:i16, "Configuration.NumCols"=w373:i16)
        n118 = Reshape Array(w376, w374, w373) -> (→"Dashboard":T1)
        n119 = call <vilib>:"Add State(s) to Queue__JKI_lib_State_Machine.vi"("State(s) in (\"\")"=w380) -> ("States Out"=w379:string)  [unwired: 14 in]
      }
      frame "--------- Event ---------" {
      }
      frame "Register User Event" {
        n120 = call "CSM - Global Log Event.vi"() -> ("error out"=w395:errorcluster, "Global Log Event"=w392:refnum<user-event>)  [unwired: 10 in]
        n121 = register-events(error in=w395, w392) -> (reference out=w394:refnum<event-registration>)  [unwired: 1 in, 1 out]
        n122 = Bundle By Name(cluster=w397, "Global Log Event"=w392) -> (w393:T8)
      }
      frame "UnRegister User Event" {
        n123 = Unregister For Events(event registration refnum=w404) -> (error out=w403:errorcluster)  [unwired: 1 in]
        n124 = Unbundle By Name(w402) -> ("Global Log Event"=w401:refnum<user-event>)
        n125 = call "CSM - Destroy Global Log Event.vi"("Error In"=w403, "CSM Global Log Event"=w401) -> ("error out"=w400:errorcluster)  [unwired: 9 in]
        n126 = call <vilib>:"Clear Errors.vi"("error in (no error)"=w400) -> ()  [unwired: 5 in, 2 out]
      }
      frame "---------- Macro ----------" {
        # "Do not put any code in this frame.\n(It is a separator no-op. You can make a copy of this frame to create a new Macro frame)"
        n127 = call <vilib>:"Add State(s) to Queue__JKI_lib_State_Machine.vi"("State(s) in (\"\")"=w413) -> ("States Out"=w412:string)  [unwired: 14 in]
      }
      frame "Macro: Initialize" {
        # "Initialization Macro\n(This is called once, when the VI starts)"
        n128 = call <vilib>:"Add State(s) to Queue__JKI_lib_State_Machine.vi"("State(s) in Front (\"\")"="Data: Initialize\nInitialize Core Data\nData: Load from INI\nUI: Initialize\nUI: Resize Dashboard\nRegister User Event\nUI: Front Panel State >> Open", "State(s) in (\"\")"=w420) -> ("States Out"=w419:string)  [unwired: 13 in]
      }
      frame "Macro: UI Refresh" {
        # "Do not put any code in this frame.\n(It is a separator no-op. You can make a copy of this frame to create a new Macro frame)"
        n129 = call <vilib>:"Add State(s) to Queue__JKI_lib_State_Machine.vi"("State(s) at Back (\"\")"="Macro: Update Terminal UI" ("State(s) in Front (\"\")")) -> ("States Out"=w425:string)  [unwired: 14 in]
        n130 = call <vilib>:"Add State(s) to Queue__JKI_lib_State_Machine.vi"("State(s) in Front (\"\")"=w425, "State(s) in (\"\")"=w428) -> ("States Out"=w427:string)  [unwired: 13 in]
      }
      frame "Macro: Update Terminal UI" {
        # "Do not put any code in this frame.\n(It is a separator no-op. You can make a copy of this frame to create a new Macro frame)"
        n131 = call <vilib>:"Add State(s) to Queue__JKI_lib_State_Machine.vi"("State(s) in Front (\"\")"="UI: Update Dashboard" ("State(s) in Front (\"\")"), "State(s) in (\"\")"=w435) -> ("States Out"=w434:string)  [unwired: 13 in]
      }
      frame "Macro: Exit" {
        # "Exit Macro\n(This is called once, when the VI exits)"
        n132 = Unbundle By Name(w445) -> ("Core.Close Panel on Exit?"=w444:bool)
        n133 = Select(t="UI: Front Panel State >> Close", s=w444, f="") -> (s? t:f=w440:string)
        n134 = call <vilib>:"Add State(s) to Queue__JKI_lib_State_Machine.vi"("State(s) in Front (\"\")"="UnRegister User Event" ("State(s) in Front (\"\")"), "State(s) in (\"\")"=w440, "State(s) at Back (\"\")"="Data: Save to INI\nData: Cleanup\nExit") -> ("States Out"=w443:string)  [unwired: 12 in]
        n135 = call <vilib>:"Add State(s) to Queue__JKI_lib_State_Machine.vi"("State(s) in Front (\"\")"=w443, "State(s) in (\"\")"=w448) -> ("States Out"=w447:string)  [unwired: 13 in]
      }
      frame "----- Action ------" {
      }
      frame "Action: Clear Non-exist JKISM" {
        n136 = Get Variant Attribute(Variant=w460) -> (duplicate Variant=w459:variant, names=w457:string[], values=w456:variant[])  [unwired: 3 in, 1 out]
        n137 = Variant To Data(type=T4[] [], Variant=w456) -> (data=w455:T4[])  [unwired: 1 in, 1 out]
        n138 = for {
          shift-right: [w476] -> w458
          shift-left: w459 -> [w477]
          tunnel: w457 -> [w475] mode=indexing
          tunnel: w455 -> [w474] mode=indexing
          n139 = Unbundle By Name(w474) -> ("Current State"=w472:string, "Name (\"\" to Use UUID)"=w471:string)
          n140 = Search 1D Array(1D array=string[] ["<Remaining States>", "Exit"], element=w472) -> (index of element=w468:i32)  [unwired: 1 in]
          n141 = Match Pattern(string=w471, regular expression="^-") -> (offset past match=w469:i32)  [unwired: 1 in, 3 out]
          n142 = Greater Or Equal To 0?(x=w468) -> (x >= 0?=w466:bool)
          n143 = Greater Or Equal To 0?(x=w469) -> (x >= 0?=w467:bool)
          n144 = Or(x=w467, y=w466) -> (x .or. y?=w465:bool)
          n145 = case shown="True" w465 {
            tunnel: w477 -> [w478 w481]
            tunnel: [w478 w480] -> w476
            tunnel: w475 -> [_ w479]
            tunnel: w471 -> [_ _]
            tunnel: w472 -> [_ _]
            frame False {
            }
            frame True {
              n146 = Delete Variant Attribute(6:w479, 7:w481) -> (3:w480:variant)  [unwired: 1 in, 2 out]
            }
          }
        }
      }
    }
  }
